vi "Initialize.vi"(8 "error in (no error)":errorcluster, 11 "CsvReportPlugin in":refnum<class "CsvReportPlugin.lvclass">) -> (0 "error out":errorcluster, 3 "CsvReportPlugin out":refnum<class "CsvReportPlugin.lvclass">)   [LabVIEW 2015, in "CsvReportPlugin.lvclass"]
uses:
  CsvReportPlugin.lvclass
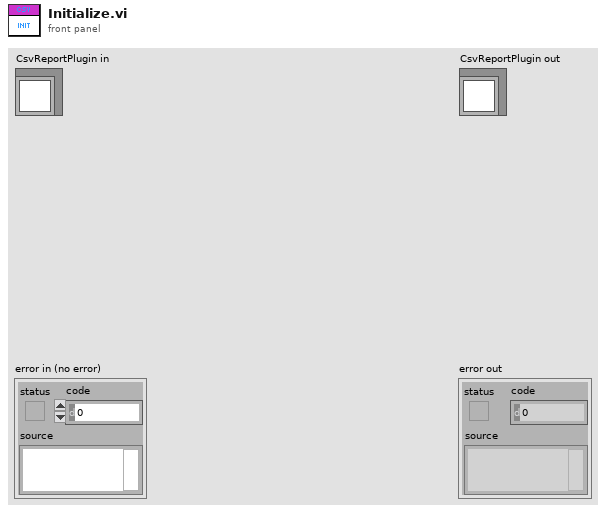
[diagram p1: front panel]
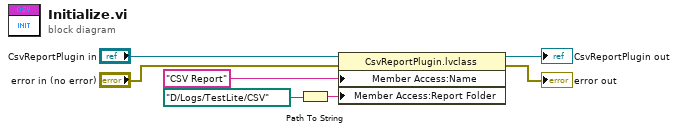
[diagram p0: block diagram]
diagram:
  n1 = Path To String(path=path "D:/Logs/TestLite/CSV" ("Report Folder")) -> (string=w1:string)
  n2 = property class="CsvReportPlugin.lvclass"(reference="CsvReportPlugin in", error in="error in (no error)", "Member Access:Name"="CSV Report" ("Name"), "Member Access:Report Folder"=w1) -> (reference out=→"CsvReportPlugin out":refnum<class "CsvReportPlugin.lvclass">, error out=→"error out":errorcluster)
